vi "Read point-to-point CSV.vi"(1 "Device Name":string="Current_PXI_1", 2 "Path":path=path "X:/Lab Configuration") -> (0 "Array Out":string[][](array[string])=[["Channel", "Channel Name", "Sensor ID", "Power Source", "Connection Diagram", "Wire Gauge", "Signaling?", "Scale", "Measurand", "Units", "Model #", "Calibration"], ["ai0", "Fuel Flow", "FM_001", "Internal", "", "", "T", "Fuel_Flow_Meter_Current_linear", "Flow", "", "", ""], ["ai1", "Water Flow", "FM_002", "Internal", "", "", "T", "Water_Flow_Meter_Current_linear", "Flow", "", "", ""], ["ai2", "Seeder Scale", "SD_001", "Internal", "", "", "T", "Seeder_Current", "Mass", "", "", ""], ["ai3", "Chamber Pressure", "TR_001", "External", "", "", "T", "Transducer_PX219-200AI_Current_linear", "Pressure", "", "", ""], ["ai4", "", "", "", "", "", "", "", "", "", "", ""], ["ai5", "", "", "", "", "", "", "", "", "", "", ""], ["ai6", "", "", "", "", "", "", "", "", "", "", ""], ["ai7", "", "", "", "", "", "", "", "", "", "", ""]])   [LabVIEW 2018]
uses:
  <vilib>/Utility/file.llb/Read Delimited Spreadsheet (string).vi
panel:
  in  "Remove rows":i32=1
  # "Overview: Demonstrates how to use the LabVIEW Report Generator Toolkit to read information from an Excel file\nRequirements: LabVIEW 2012 Base Development System (or compatible)\n                             LabVIEW 2012 Report Generation Toolkit (or compatible)\n                             Microsoft Excel\n                             (KB 3EJEC9NS: Report Generation Toolkit Compatibility with Microsoft Office and LabVIEW\n                             http://digital.ni.com/public.nsf/allkb/C9408B9F08D711E786256F3300701D01)\nInstructions: \n1. Run the VI"
  # "Sheet 3"
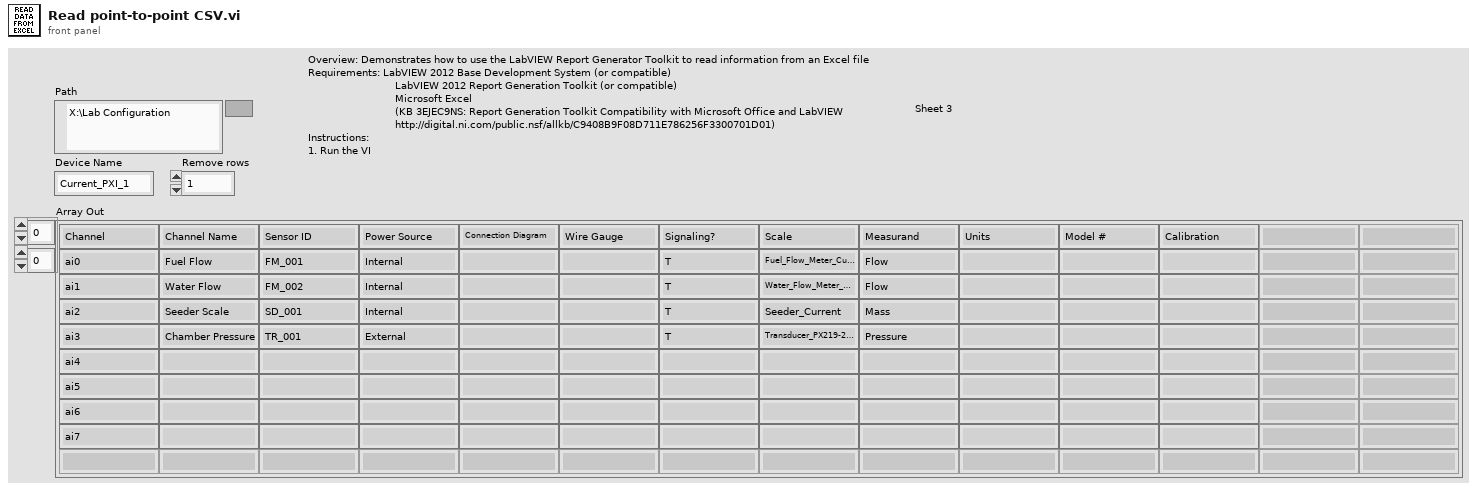
[diagram p1: front panel]
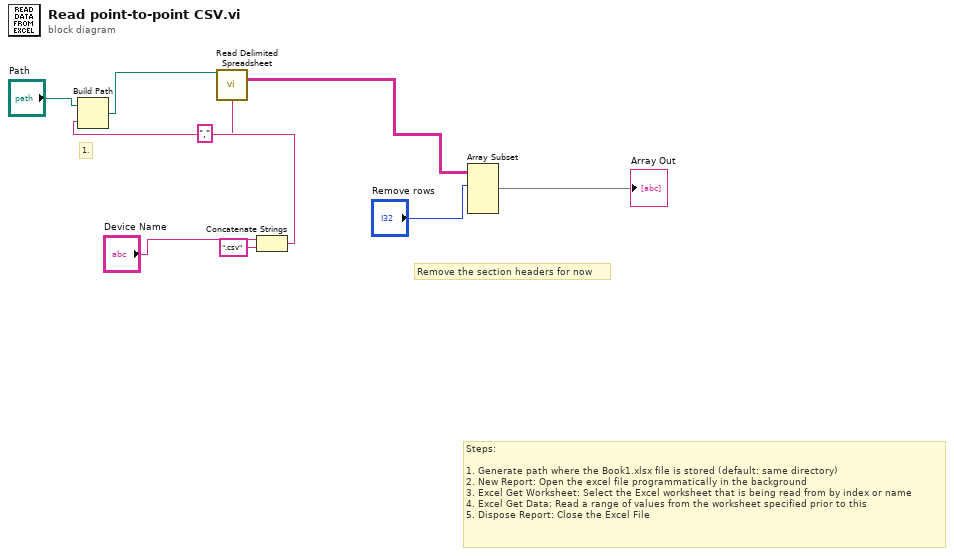
[diagram p0: block diagram]
diagram:
  # "Remove the section headers for now"
  # "1."
  # "Steps:\n\n1. Generate path where the Book1.xlsx file is stored (default: same directory)\n2. New Report: Open the excel file programmatically in the background\n3. Excel Get Worksheet: Select the Excel worksheet that is being read from by index or name\n4. Excel Get Data: Read a range of values from the worksheet specified prior to this\n5. Dispose Report: Close the Excel File"
  n1 = Concatenate Strings("Device Name", ".csv" ("string")) -> (w4:string)
  n2 = Build Path(base path="Path", name or relative path=w4) -> (appended path=w3:path)
  n3 = call-poly <vilib>:"Read Delimited Spreadsheet.vi"("file path (dialog if empty)"=w3, "delimiter (\\t)"="," ("delimiter (\\t)")) -> ("all rows"=w2:string[][])  [unwired: 8 in, 5 out]
  n4 = Array Subset(array=w2, index (row)="Remove rows") -> (→"Array Out":string[][])  [unwired: 3 in]
